vi "TCP Close.vi"(8 "Error In":errorcluster, 11 "LINX Decice Config":T1) -> (0 "Error Out":errorcluster, 3 "LINX Decice Config":T1)   [LabVIEW 2018, in "LVH-LINX.lvlib" / "Device.lvlib"]
uses:
  Device.lvlib
  Type Defs/LINX Device Config.ctl
  Type Defs/Interface.ctl
  Type Defs/TCP Config.ctl
  Type Defs/Device Family.ctl
  LVH-LINX.lvlib
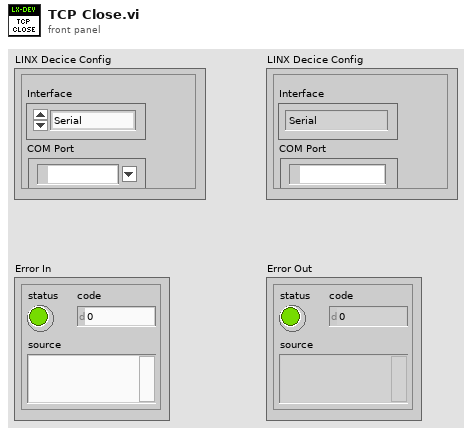
[diagram p1: front panel]
types:
  T1 = typedef "LVH-LINX.lvlib/Device.lvlib/LINX Device Config.ctl" = cluster{"Interface":T2, "COM Port":refnum<visa-resource-name>, "TCP Configuration":T3, "Device Family":T4, "Device ID":u8, "Device Name":string, "TCP Ref":refnum<k5>}
  T2 = typedef "LVH-LINX.lvlib/Interface.ctl" = enum16{"Serial", "TCP"}
  T3 = typedef "LVH-LINX.lvlib/Device.lvlib/TCP Config.ctl" = cluster{"IP Address":string, "Port":u16}
  T4 = typedef "LVH-LINX.lvlib/Device Family.ctl" = enum8{"National Instruments", "Digilent", "Arduino"}
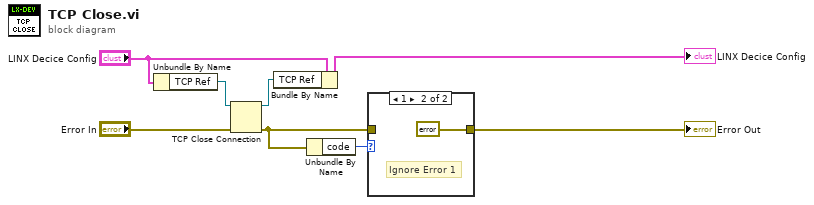
[diagram p0: block diagram]
diagram:
  n1 = Unbundle By Name("LINX Decice Config") -> ("TCP Ref"=w8:refnum<k5>)
  n2 = TCP Close Connection(connection ID=w8, error in (no error)="Error In") -> (connection ID out=w6:refnum<k5>, error out=w1:errorcluster)  [unwired: 1 in]
  n3 = Bundle By Name(cluster="LINX Decice Config", "TCP Ref"=w6) -> (→"LINX Decice Config":T1)
  n4 = Unbundle By Name(w1) -> ("code"=w3:i32)
  n5 = case shown="1" w3 {
    tunnel: [w9 errorcluster {"status"=FALSE, "code"=0, "source"=""} ("error out")] -> w2
    tunnel: w1 -> [w9 _]
    frame 0, Default {
    }
    frame 1 {
      # "Ignore Error 1"
    }
  }
  "Error Out" <- w2
